vi "Release Tree Manager.vi"(8 "Error In":errorcluster, 11 "Tree Manager":T1) -> (0 "Error Out":errorcluster)   [LabVIEW 2016, in "Tree Manager.lvclass"]
doc: "Releases an obtained reference to the Tree Manager."
uses:
  Tree Manager.lvclass
  Typedefs/Session Handle.ctl
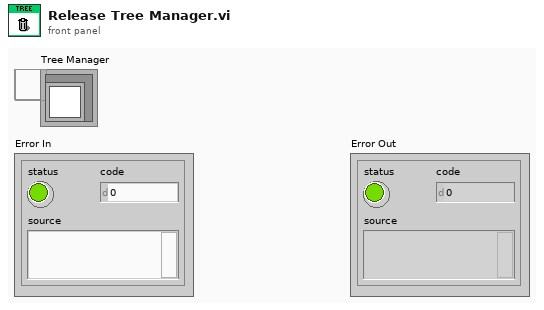
[diagram p1: front panel]
types:
  T1 = typedef "Tree Manager.lvclass/Session Handle.ctl" = refnum<data-value>
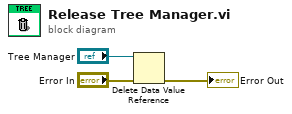
[diagram p0: block diagram]
diagram:
  n1 = Delete Data Value Reference(data value reference="Tree Manager", error in="Error In") -> (error out=→"Error Out":errorcluster)  [unwired: 1 out]
